vi "CurrencyConverter.vi"() -> ()   [LabVIEW 2016]
uses:
  <vilib>/express/express arith-compare/Formula/XNode/ExpressFormulaBlockNode.xnode
panel:
  in  "New Currency In":string(combo)
  out "New Currency Out":string
  out "Money in":dbl
  in  "Money in USD":dbl
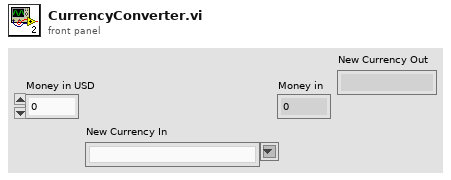
[diagram p1: front panel]
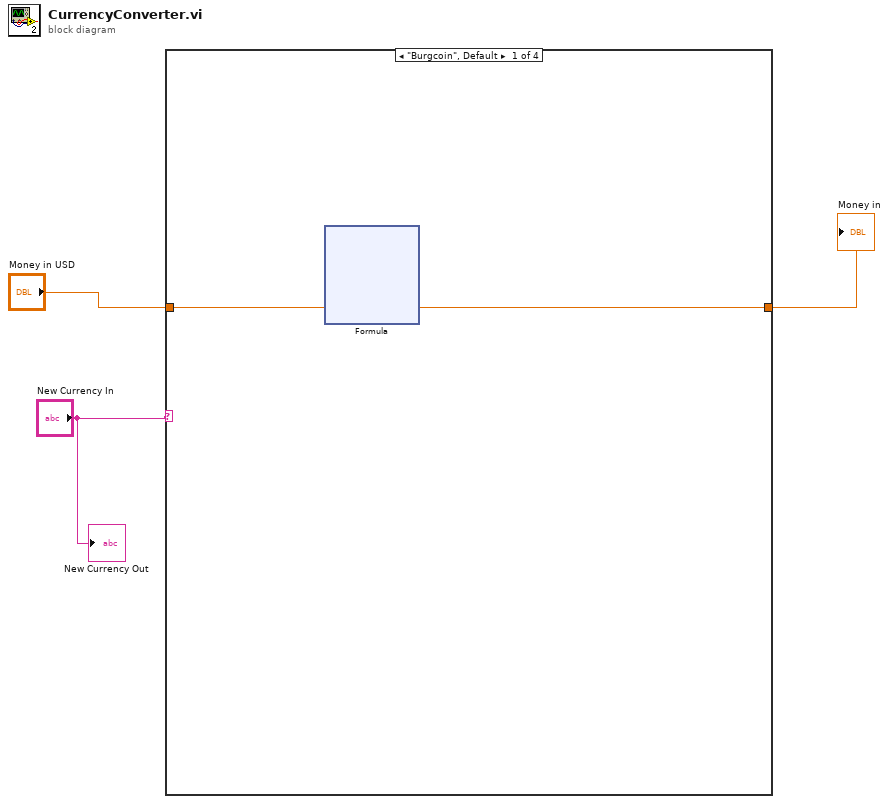
[diagram p0: block diagram]
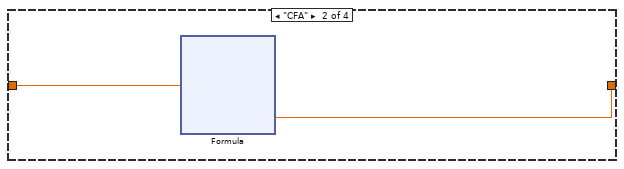
[diagram p2: hidden frame]
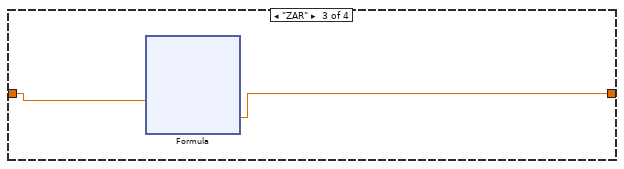
[diagram p3: hidden frame]
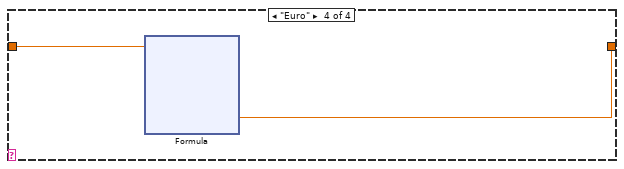
[diagram p4: hidden frame]
diagram:
  n1 = case shown="\"Burgcoin\", Default" "New Currency In" {
    tunnel: "Money in USD" -> [w5 w15 w25 w35]
    tunnel: [w4 w14 w24 w34] -> w2
    frame "Burgcoin", Default {
      n2 = xnode "Formula"("m"=w5) -> ("Result"=w4:dbl)  [unwired: 1 in, 1 out]
    }
    frame "CFA" {
      n3 = xnode "Formula"("m"=w15) -> ("Result"=w14:dbl)  [unwired: 1 in, 1 out]
    }
    frame "ZAR" {
      n4 = xnode "Formula"("m"=w25) -> ("Result"=w24:dbl)  [unwired: 1 in, 1 out]
    }
    frame "Euro" {
      n5 = xnode "Formula"("m"=w35) -> ("Result"=w34:dbl)  [unwired: 1 in, 1 out]
    }
  }
  "Money in" <- w2
  "New Currency Out" <- "New Currency In"
